vi "FieldRenderer.vi"(1 "FirstCall?":bool=TRUE, 2 "FieldLength":i32, 3 "FieldArray":T1[][](array[typedef])) -> (0 "FieldDisplay":picture)   [LabVIEW 2025]
uses:
  common/types/network/FoggedFieldCell.ctl
  server/types/TerrainEnum.ctl
  af7561f3-d307-47ef-bb87-90422b90b63f.vi
  ClientGlobalVariables.vi
  <vilib>/Dataflow_G/G-Image/Image Processing/Polymorphic VIs/Resize Image (WxH).vi
  <vilib>/picture/picture.llb/Draw True-Color Pixmap.vi
  <vilib>/Dataflow_G/G-Image/G-Image.lvlib
panel:
  out "LastFieldArray":T1[][](array[typedef])
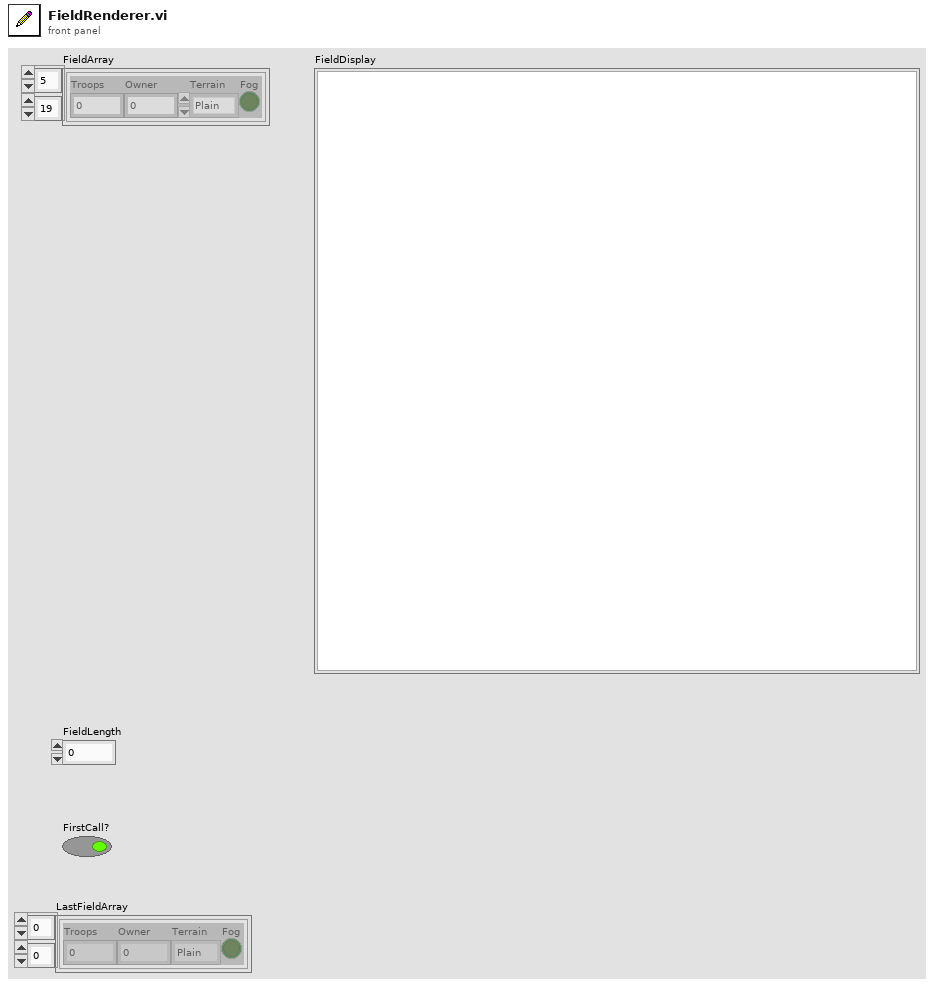
[diagram p1: front panel]
types:
  T1 = typedef "FoggedFieldCell.ctl" = cluster{"Troops":u32, "Owner":i32, "Terrain":T2, "Fog":bool}
  T2 = typedef "TerrainEnum.ctl" = enum16{"Plain", "Mountain", "City", "General"}
  T3 = typedef "imagedata.ctl" = cluster{"image type":i32, "image depth":i32, "image":u8[], "mask":u8[], "colors":u32[], "Rectangle":cluster{"left":i16, "top":i16, "right":i16, "bottom":i16}}
  T4 = cluster{"left":i16, "top":i16, "right":i16, "bottom":i16}
  T5 = cluster{"Font Name:":string, "Size":i16, "Strikeout?":bool, "Italic?":bool, "Underline?":bool, "Outline?":bool, "Shadow?":bool, "Bold?":bool}
  T6 = cluster{"horizontal":enum16{"left", "center", "right"}, "vertical":enum16{"top", "center", "bottom"}}
  T7 = cluster{"Troops":bool, "Owner":bool, "Terrain":bool, "Fog":bool}
  T8 = map{u32, cluster{"Name":string, "Team":u8, "Ready":bool, "Host":bool, "Alive":bool, "Color":u32, "Lands":set{cluster{"Row":u32, "Column":u32}}, "Army":u32}}
  T9 = cluster{"Name":string, "Team":u8, "Ready":bool, "Host":bool, "Alive":bool, "Color":u32, "Lands":set{cluster{"Row":u32, "Column":u32}}, "Army":u32}
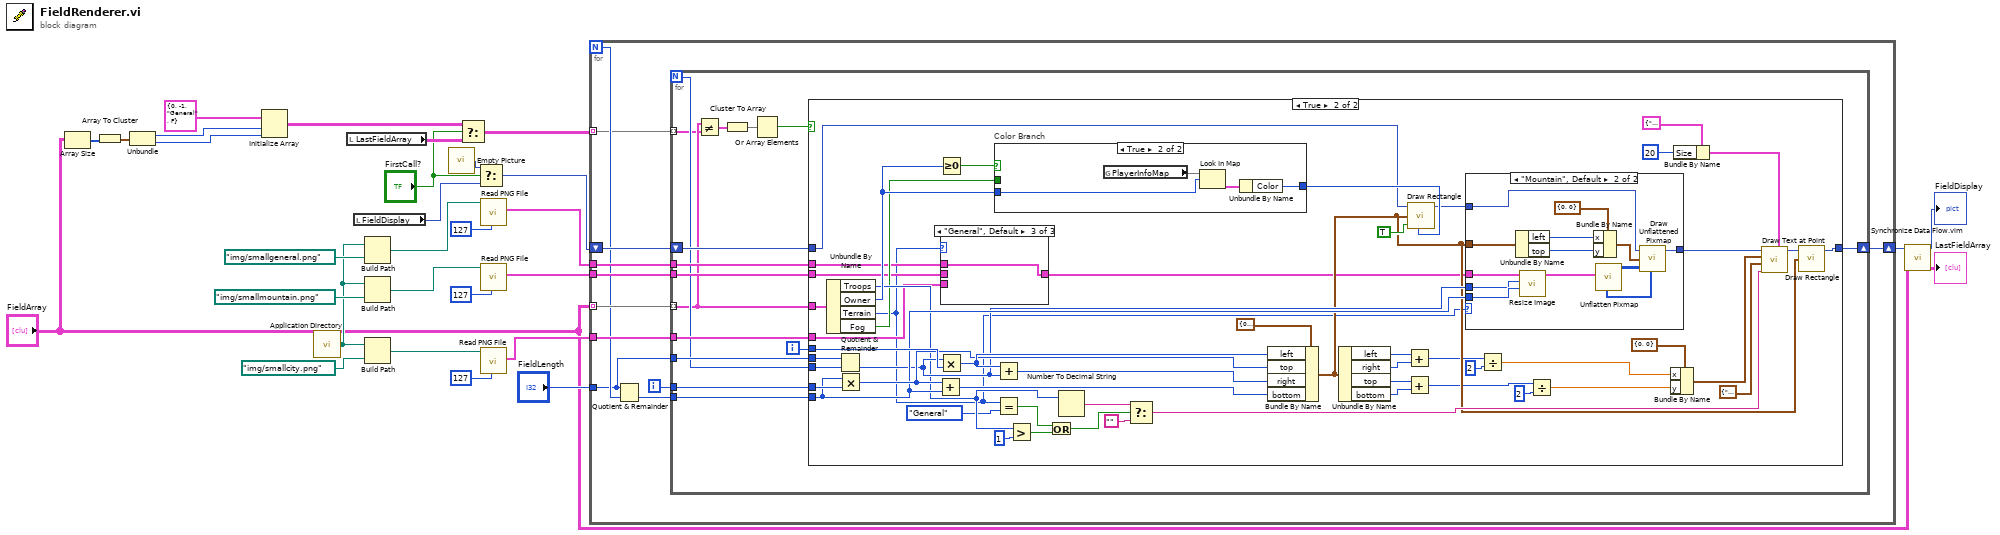
[diagram p0: block diagram]
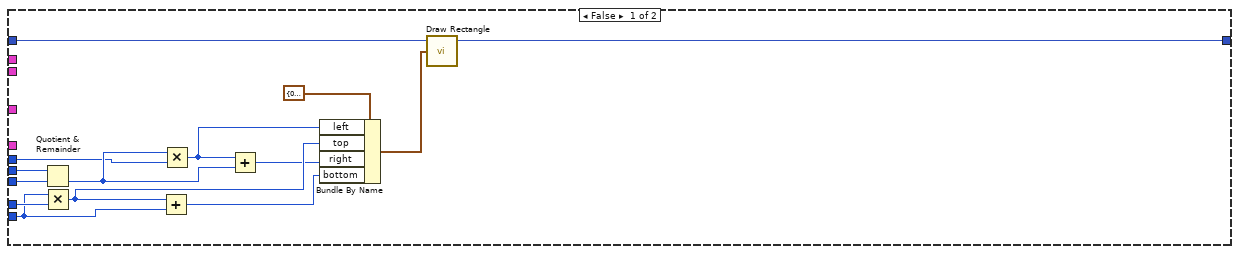
[diagram p2: hidden frame]
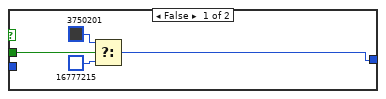
[diagram p6: hidden frame]
diagram:
  n1 = Array Size(array="FieldArray") -> (size(s)=w10:i32[])
  n2 = Array To Cluster(array=w10) -> (cluster=w9:cluster{"[0]":i32, "[1]":i32})
  n3 = Unbundle(w9) -> ("[0]"=w8:i32, "[1]"=w7:i32)
  n4 = Initialize Array(T1 {"Troops"=0, "Owner"=-1, "Terrain"=enum."General", "Fog"=FALSE} ("CellInfo 2"), w8, w7) -> (w11:T1[][])
  n5 = call <vilib>:"Application Directory.vi"() -> ("Application Directory"=w18:path)
  n6 = local read "LastFieldArray"() -> (w3:T1[][])
  n7 = local read "FieldDisplay"() -> (w5:picture)
  n8 = Build Path(base path=w18, name or relative path=path "img/smallgeneral.png" ("path to PNG file")) -> (appended path=w29:path)
  n9 = Build Path(base path=w18, name or relative path=path "img/smallmountain.png" ("path to PNG file")) -> (appended path=w28:path)
  n10 = Build Path(base path=w18, name or relative path=path "img/smallcity.png" ("path to PNG file")) -> (appended path=w30:path)
  n11 = call "Empty Picture"() -> ("empty picture"=w14:picture)
  n12 = Select(t=w11, s="FirstCall?", f=w3) -> (s? t:f=w13:T1[][])
  n13 = Select(t=w14, s="FirstCall?", f=w5) -> (s? t:f=w15:picture)
  n14 = call <vilib>:"Read PNG File.vi"("Transparency Thresh"=u8 127, "path to PNG file"=w29) -> ("image data"=w21:T3)  [unwired: 7 in, 2 out]
  n15 = call <vilib>:"Read PNG File.vi"("Transparency Thresh"=u8 127, "path to PNG file"=w28) -> ("image data"=w19:T3)  [unwired: 7 in, 2 out]
  n16 = call <vilib>:"Read PNG File.vi"("Transparency Thresh"=u8 127, "path to PNG file"=w30) -> ("image data"=w20:T3)  [unwired: 7 in, 2 out]
  n17 = for {
    N -> [w34]
    shift-right: [w40] -> w16
    shift-left: w15 -> [w41]
    tunnel: "FieldArray" -> [w39] mode=indexing
    tunnel: w20 -> [w37]
    tunnel: w21 -> [w36]
    tunnel: w19 -> [w35]
    tunnel: "FieldLength" -> [w31]
    tunnel: w13 -> [w32] mode=indexing
    i -> [w38]
    n18 = Quotient & Remainder(x=w31, y=w34) -> (floor(x/y)=w33:i32)  [unwired: 1 out]
    n19 = for {
      N -> [w47]
      shift-right: [w53] -> w40
      shift-left: w41 -> [w54]
      tunnel: w39 -> [w46] mode=indexing
      tunnel: w38 -> [w56]
      tunnel: w33 -> [w52]
      tunnel: w37 -> [w50]
      tunnel: w36 -> [w51]
      tunnel: w35 -> [w49]
      tunnel: w31 -> [w48]
      tunnel: w32 -> [w42] mode=indexing
      i -> [w55]
      n20 = Not Equal?(x=w46, y=w42) -> (x != y?=w44:T7)
      n21 = Cluster To Array(cluster=w44) -> (array=w45:bool[])
      n22 = Or Array Elements(Boolean array=w45) -> (logical OR=w43:bool)
      n23 = case shown="True" w43 {
        tunnel: w56 -> [w63 w123]
        tunnel: w55 -> [w64 w122]
        tunnel: w54 -> [w59 w111]
        tunnel: [w60 w109] -> w53
        tunnel: w52 -> [w61 w108]
        tunnel: w51 -> [_ w82]
        tunnel: w50 -> [_ w84]
        tunnel: w49 -> [_ w83]
        tunnel: w48 -> [w62 w105]
        tunnel: w47 -> [w57 w104]
        tunnel: w46 -> [_ w86]
        frame False {
          n24 = Quotient & Remainder(x=w62, y=w57) -> (floor(x/y)=w65:i32)  [unwired: 1 out]
          n25 = Multiply(x=w61, y=w63) -> (x*y=w68:i32)
          n26 = Add(x=w68, y=w61) -> (x+y=w67:i32)
          n27 = Multiply(x=w65, y=w64) -> (x*y=w69:i32)
          n28 = Add(x=w69, y=w65) -> (x+y=w66:i32)
          n29 = Bundle By Name(cluster=T4 {"left"=0, "top"=0, "right"=0, "bottom"=0} ("rect"), "left"=w69, "top"=w68, "right"=w66, "bottom"=w67) -> (w58:T4)
          n30 = call <vilib>:"Draw Rectangle.vi"("picture"=w59, "rect"=w58) -> ("new picture"=w60:picture)  [unwired: 7 in]
        }
        frame True {
          n31 = Unbundle By Name(w86) -> ("Troops"=w88:u32, "Owner"=w118:i32, "Terrain"=w76:T2, "Fog"=w85:bool)
          n32 = Quotient & Remainder(x=w105, y=w104) -> (floor(x/y)=w103:i32)  [unwired: 1 out]
          n33 = Multiply(x=w108, y=w123) -> (x*y=w115:i32)
          n34 = Add(x=w115, y=w108) -> (x+y=w114:i32)
          n35 = Greater Or Equal To 0?(x=w118) -> (x >= 0?=w119:bool)
          n36 = Multiply(x=w103, y=w122) -> (x*y=w116:i32)
          n37 = case shown="\"General\", Default" w76 {
            tunnel: w84 -> [_ w125 _]
            tunnel: w83 -> [w124 _ _]
            tunnel: w82 -> [_ _ w126]
            tunnel: [w124 w125 w126] -> w81
            frame "Mountain" {
            }
            frame "City" {
            }
            frame "General", Default {
            }
          }
          n38 = case "Color Branch" shown="True" w119 {
            tunnel: w118 -> [_ w148]
            tunnel: [w144 w146] -> w112
            tunnel: w85 -> [w143 _]
            frame False {
              n39 = Select(t=u32 3750201, s=w143, f=u32 16777215) -> (s? t:f=w144:u32)
            }
            frame True {
              n40 = global read "ClientGlobalVariables.vi" "PlayerInfoMap"() -> (w145:T8)
              n41 = Look In Map(map=w145, key=w148) -> (value=w147:T9)  [unwired: 1 in, 1 out]
              n42 = Unbundle By Name(w147) -> ("Color"=w146:u32)
            }
          }
          n43 = Add(x=w116, y=w103) -> (x+y=w113:i32)
          n44 = Equal?(x=w76, y=TerrainEnum."General") -> (x = y?=w73:bool)
          n45 = Greater?(x=w88, y=u32 1) -> (0:w77:bool)
          n46 = Or(x=w73, y=w77) -> (x .or. y?=w74:bool)
          n47 = Number To Decimal String(number=w88) -> (decimal integer string=w72:string)  [unwired: 1 in]
          n48 = Select(t=w72, s=w74, f="") -> (s? t:f=w117:string)
          n49 = Bundle By Name(cluster=T4 {"left"=0, "top"=0, "right"=0, "bottom"=0} ("rect"), "left"=w116, "top"=w115, "right"=w113, "bottom"=w114) -> (w102:T4)
          n50 = Unbundle By Name(w102) -> ("left"=w101:i16, "right"=w100:i16, "top"=w95:i16, "bottom"=w94:i16)
          n51 = Add(x=w101, y=w100) -> (x+y=w99:i16)
          n52 = Add(x=w95, y=w94) -> (x+y=w97:i16)
          n53 = call <vilib>:"Draw Rectangle.vi"("picture"=w111, "rect"=w102, "fill?(F)"=TRUE, "color(black)"=w112) -> ("new picture"=w107:picture)  [unwired: 5 in]
          n54 = case shown="\"Mountain\", Default" w76 {
            tunnel: w108 -> [_ w140]
            tunnel: w103 -> [_ w139]
            tunnel: w107 -> [w127 w131]
            tunnel: [w127 w130] -> w106
            tunnel: w102 -> [_ w137]
            tunnel: w81 -> [_ w128]
            frame "Plain" {
            }
            frame "Mountain", Default {
              n55 = Unbundle By Name(w137) -> ("left"=w135:i16, "top"=w134:i16)
              n56 = call-poly <vilib>:"Resize Image.vi"("Height"=w140, "Width"=w139, "Image"=w128) -> ("Resized Image"=w138:T3)  [unwired: 7 in, 1 out]
              n57 = Bundle By Name(cluster=cluster{"x":i16, "y":i16} {"x"=0, "y"=0} ("top left point(0, 0)"), "x"=w135, "y"=w134) -> (w133:cluster{"x":i16, "y":i16})
              n58 = call <vilib>:"Unflatten Pixmap.vi"("image data"=w138) -> ("24-bit pixmap"=w132:u32[][], "mask"=w129:u8[])  [unwired: 4 in, 5 out]
              n59 = call-poly <vilib>:"Draw Unflattened Pixmap.vi"("picture"=w131, "top left point(0, 0)"=w133, "data (RGB format)"=w132, "mask"=w129) -> ("new picture"=w130:picture)  [unwired: 5 in]
            }
          }
          n60 = Divide(x=w99, y=i16 2) -> (x/y=w91:dbl)
          n61 = Divide(x=w97, y=i16 2) -> (x/y=w90:dbl)
          n62 = Bundle By Name(cluster=cluster{"x":i16, "y":i16} {"x"=0, "y"=0} ("origin"), "x"=w91, "y"=w90) -> (w89:cluster{"x":i16, "y":i16})
          n63 = Bundle By Name(cluster=T5 {"Font Name:"="", "Size"=12, "Strikeout?"=FALSE, "Italic?"=FALSE, "Underline?"=FALSE, "Outline?"=FALSE, "Shadow?"=FALSE, "Bold?"=FALSE} ("[user-specified font]"), "Size"=i16 20) -> (w78:T5)
          n64 = call <vilib>:"Draw Text at Point.vi"("[user-specified font]"=w78, "text"=w117, "alignment(left, top)"=T6 {"horizontal"=enum."center", "vertical"=enum."center"}, "origin"=w89, "picture"=w106) -> ("new picture"=w110:picture)  [unwired: 5 in, 1 out]
          n65 = call <vilib>:"Draw Rectangle.vi"("picture"=w110, "rect"=w102) -> ("new picture"=w109:picture)  [unwired: 7 in]
        }
      }
    }
  }
  n66 = call "Synchronize Data Flow.vim"("input 4"="FieldArray", "input 1"=w16) -> ("output 4"=→"LastFieldArray":T1[][], "output 1"=→"FieldDisplay":picture)  [unwired: 2 in, 2 out]
